vi "Queue Nested Status.vi"(11 "Base Queue jettl in":refnum<class "Base Queue jettl.lvclass">) -> (0 "Queue Nested Count":i32, 1 "Queue Nested Aliases":string[](array[string]), 2 "Any Exist?":bool, 3 "Base Queue jettl out":refnum<class "Base Queue jettl.lvclass">)   [LabVIEW 2021, in "jettl.lvlib" / "Base Queue jettl.lvlib" / "Base Queue jettl.lvclass"]
uses:
  Base Queue jettl.lvclass
  C:/git/jettl/src/jettl/jettl/jettl.lvclass
  Base Queue jettl.lvclass/Base Queue jettl.ctl
  jettl/jettl.lvclass
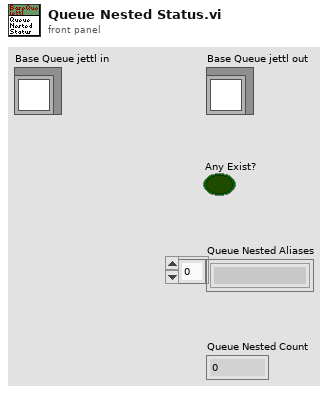
[diagram p1: front panel]
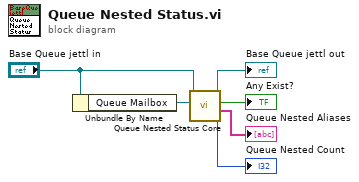
[diagram p0: block diagram]
diagram:
  n1 = Unbundle By Name("Base Queue jettl in") -> ("Queue Mailbox"=w6:refnum<data-value>)
  n2 = call "Queue Nested Status Core.vi"("Queue Mailbox"=w6, "jettl in"="Base Queue jettl in") -> ("Queue Nested Count"=→"Queue Nested Count":i32, "Queue Nested Aliases"=→"Queue Nested Aliases":string[], "Any Exist?"=→"Any Exist?":bool, "jettl out"=→"Base Queue jettl out":refnum<class "Base Queue jettl.lvclass">)  [unwired: 6 in]
